vi "KEYSIGHT_DSO3034G_scope.vi"() -> ()   [LabVIEW 2026]
uses:
  <vilib>/wsapi/NI_WebServices.lvlib
panel:
  out "scope path":path
  out "2D Picture 2":picture
  in  "write buffer":string=":DISPlay:DATA? PNG, COLOR"
  in  "VISA resource name":refnum<visa-resource-name>
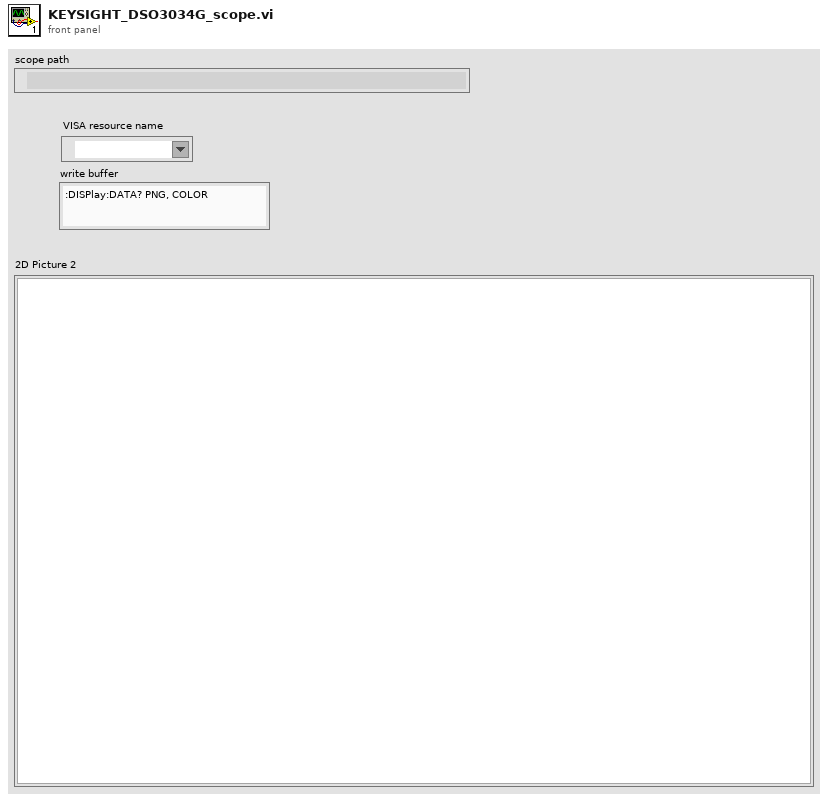
[diagram p1: front panel]
types:
  T1 = typedef "imagedata.ctl" = cluster{"image type":i32, "image depth":i32, "image":u8[], "mask":u8[], "colors":u32[], "Rectangle":cluster{"left":i16, "top":i16, "right":i16, "bottom":i16}}
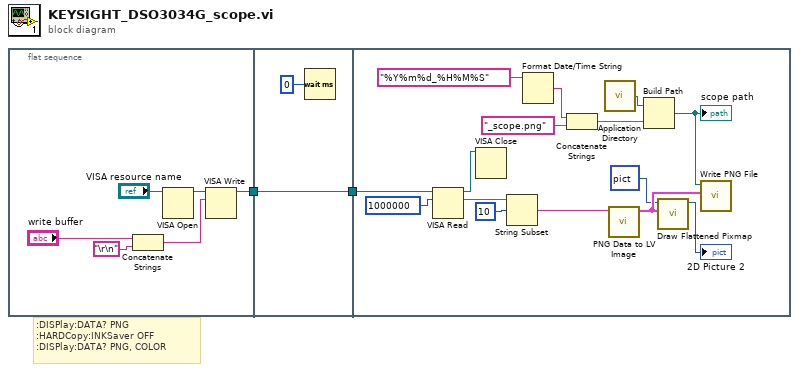
[diagram p0: block diagram]
diagram:
  # ":DISPlay:DATA? PNG\n:HARDCopy:INKSaver OFF\n:DISPlay:DATA? PNG, COLOR"
  n1 = flat-sequence {
    tunnel: [w3] -> w2
    tunnel: w2 -> [w9]
    tunnel: [w9] -> w1
    tunnel: w1 -> [w24]
    frame #0 {
      n2 = Concatenate Strings("write buffer", "\r\n") -> (w4:string)
      n3 = VISA Open(VISA resource name="VISA resource name") -> (VISA resource name=w7:refnum<visa-resource-name>)  [unwired: 4 in, 1 out]
      n4 = VISA Write(VISA resource name=w7, write buffer=w4) -> (VISA resource name out=w3:refnum<visa-resource-name>)  [unwired: 1 in, 2 out]
    }
    frame #1 {
      n5 = Wait (ms)(milliseconds to wait=u32 0) -> ()  [unwired: 1 out]
    }
    frame #2 {
      n6 = VISA Read(VISA resource name=w24, byte count=u32 1000000) -> (VISA resource name out=w17:refnum<visa-resource-name>, read buffer=w18:string)  [unwired: 1 in, 2 out]
      n7 = VISA Close(VISA resource name=w17) -> ()  [unwired: 1 in, 1 out]
      n8 = String Subset(string=w18, offset (0)=10) -> (substring=w21:string)  [unwired: 1 in]
      n9 = Format Date/Time String(time format string (%c)="%Y%m%d_%H%M%S") -> (date/time string=w14:string)  [unwired: 2 in]
      n10 = Concatenate Strings(w14, "_scope.png") -> (w11:string)
      n11 = call <vilib>:"Application Directory.vi"() -> ("Application Directory"=w15:path)
      n12 = call <vilib>:"PNG Data to LV Image.vi"("png data"=w21) -> ("image data"=w23:T1)  [unwired: 9 in, 1 out]
      n13 = Build Path(base path=w15, name or relative path=w11) -> (appended path=w16:path)
      "scope path" <- w16
      n14 = call <vilib>:"Draw Flattened Pixmap.vi"("image data"=w23, "picture"=picture data[5B]) -> ("new picture"=→"2D Picture 2":picture)  [unwired: 7 in]
      n15 = call <vilib>:"Write PNG File.vi"("image data"=w23, "path to PNG file"=w16) -> ()  [unwired: 8 in, 2 out]
    }
  }
